vi "DatabaseTest.vi"(3 "error in (no error)":errorcluster) -> (0 "error out":errorcluster, 2 "数据库连接成功":bool)   [LabVIEW 2019]
uses:
  <vilib>/Utility/error.llb/DialogType.ctl
  <vilib>/addons/database/Connection.llb/DB Tools Open Connec (String).vi
  <vilib>/addons/database/NI_Database_API.lvlib
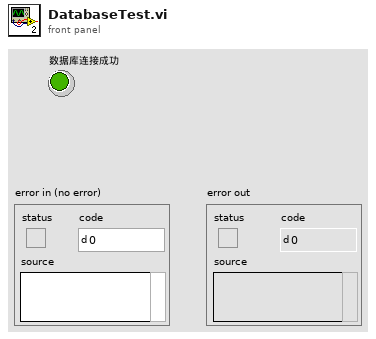
[diagram p1: front panel]
types:
  T1 = typedef "DialogType.ctl" = u16
  T2 = typedef "NI_Database_API.lvlib/Conn ObjectReference.ctl" = refnum<k1>
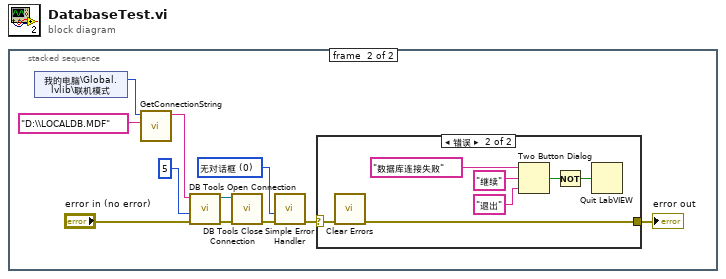
[diagram p0: block diagram]
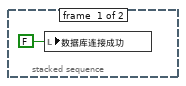
[diagram p2: hidden frame]
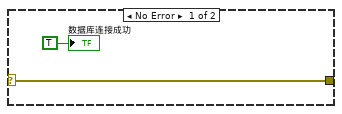
[diagram p3: hidden frame]
diagram:
  n1 = stacked-sequence {
    frame #0 {
      n2 = local write "数据库连接成功"(FALSE ("数据库连接成功")) -> ()
    }
    frame #1 {
      w8 = T1 0 items=["无对话框", "确定信息", "继续或停止信息", "确定信息＋警告", "继续/停止+警告"] ("type of dialog (OK msg:1)")
      n3 = shared-variable "我的电脑\\Global.lvlib\\联机模式"() -> (w2:i16)  [unwired: 1 in, 1 out]
      n4 = call "GetConnectionString.vi"("Database Name"="D:\\LOCALDB.MDF", "连接模式"=w2) -> ("连接字符串"=w5:string)  [unwired: 4 in, 1 out]
      n5 = call-poly <vilib>:"DB Tools Open Connection.vi"("error in (no error)"="error in (no error)", "connection timeout (15)"=5, "connection information"=w5) -> ("error out"=w12:errorcluster, "connection reference"=w11:T2)  [unwired: 5 in]
      n6 = call <vilib>:"DB Tools Close Connection.vi"("error in (no error)"=w12, "connection reference"=w11) -> ("error out"=w9:errorcluster)  [unwired: 5 in]
      n7 = call <vilib>:"Simple Error Handler.vi"("type of dialog (OK msg:1)"=w8, "error in (no error)"=w9) -> ("error out"=w4:errorcluster)  [unwired: 3 in, 4 out]
      n8 = case shown="错误" w4 {
        selector: w4 -> [w13 w16]
        tunnel: [w13 w15] -> w3
        frame No Error {
          "数据库连接成功" <- TRUE ("数据库连接成功")
        }
        frame Error {
          n9 = call <vilib>:"Clear Errors.vi"("error in (no error)"=w16) -> ("error out"=w15:errorcluster)  [unwired: 5 in, 1 out]
          n10 = Two Button Dialog(message="数据库连接失败" ("消息"), 1:"退出" ("F按钮名称（“取消”）"), 2:"继续" ("T按钮名称（“确定”）")) -> (T button?=w18:bool)
          n11 = Not(x=w18) -> (.not. x?=w17:bool)
          n12 = Quit LabVIEW(quit? (T)=w17) -> ()
        }
      }
      "error out" <- w3
    }
  }
